vi "EditRowValue.vi"(0 "VI Reference In":refnum<vi>, 2 "delimiter (>>)":string=">>", 5 "Control Path":string, 7 "Row Index":i32, 9 "Value":string[](array[string]), 11 "Error In":errorcluster) -> (4 "VI Reference Out":refnum<vi>, 15 "Error Out":errorcluster)   [LabVIEW 2016, in "Drona.lvlib" / "ControlValue.lvlib" / "StimulusTable.lvlib"]
doc: "Sets value(signaling) for the table control whose row index is specified. \n\nThe input control name is given as a string , incase of path, use delimiters inbetween the path."
uses:
  StimulusTable.lvlib
  <vilib>/Utility/error.llb/Error Cluster From Error Code.vi
  <vilib>/ErrorRing/Error Ring.xnode
  Drona.lvlib
  Get/GetControlRef/GetControlRef.lvlib
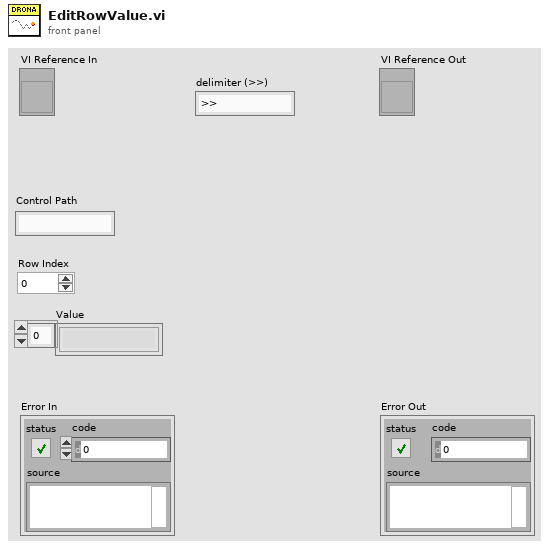
[diagram p1: front panel]
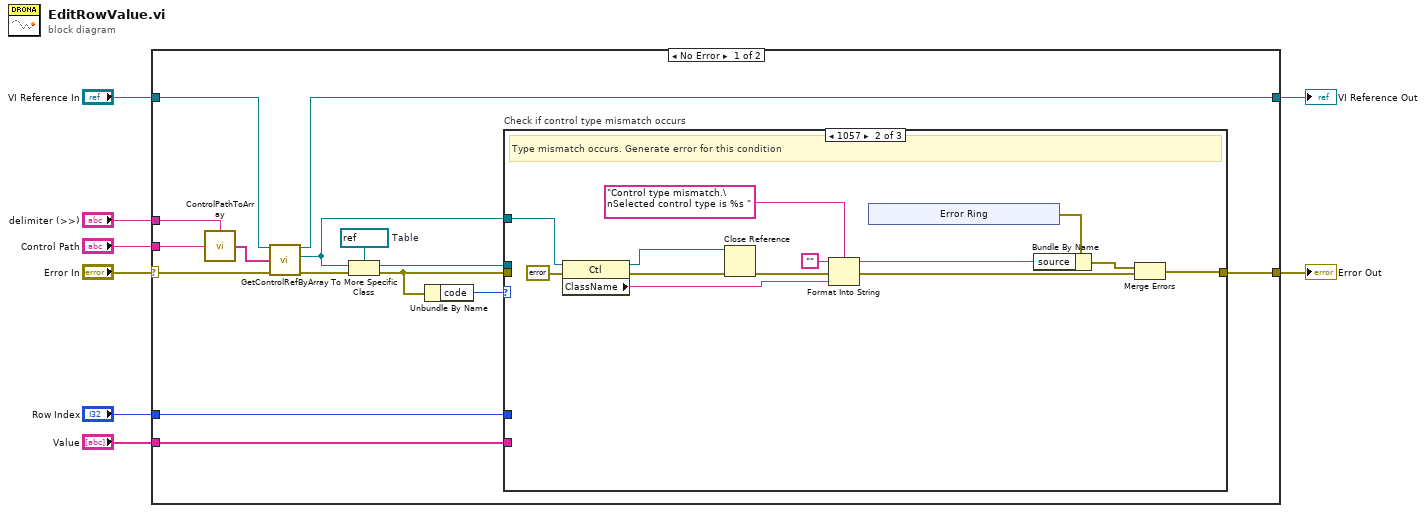
[diagram p0: block diagram]
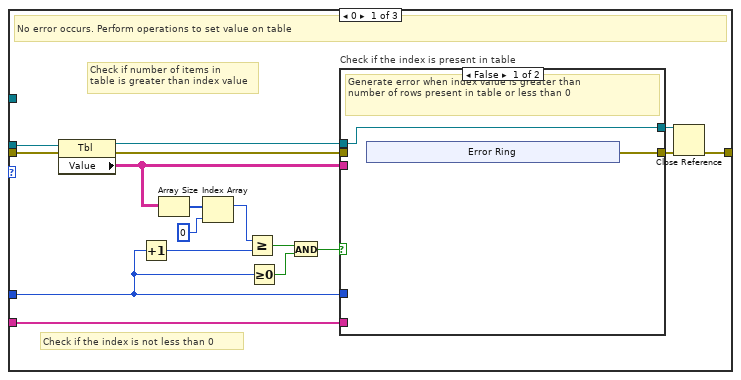
[diagram p2: hidden frame]
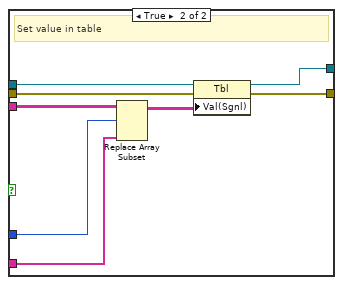
[diagram p3: hidden frame]
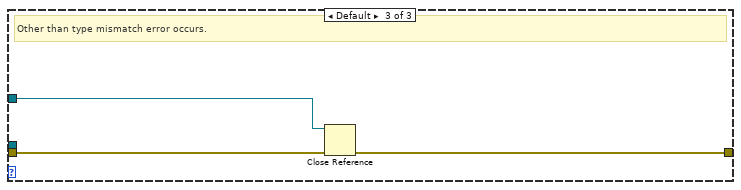
[diagram p4: hidden frame]
diagram:
  n1 = case shown="No Error" "Error In" {
    selector: "Error In" -> [w12 w78]
    tunnel: [w20 w78] -> w7
    tunnel: "VI Reference In" -> [w16 w77]
    tunnel: "Control Path" -> [w22 _]
    tunnel: "Row Index" -> [w18 _]
    tunnel: [w15 w77] -> w3
    tunnel: "delimiter (>>)" -> [w21 _]
    tunnel: "Value" -> [w9 _]
    frame No Error {
      w23 = refnum<vi> refnum  # Table
      n2 = call "ControlPathToArray.vi"("Control Name"=w22, "delimiter (>>)"=w21) -> ("Control Path"=w17:string[])
      n3 = call "GetControlRefByArray.vi"("VI Reference In"=w16, "Control Path"=w17, "error In"=w12) -> ("VI Reference Out"=w15:refnum<vi>, "Ctl Refnum"=w13:refnum<vi>, "error out"=w14:errorcluster)  [unwired: 10 in]
      n4 = To More Specific Class(target class=w23, reference=w13, error in=w14) -> (specific class reference=w19:refnum<vi>, error out=w11:errorcluster)
      n5 = Unbundle By Name(w11) -> ("code"=w10:i32)
      n6 = case "Check if control type mismatch occurs" shown="1057" w10 {
        tunnel: [w40 w58 w75] -> w20
        tunnel: w19 -> [w33 _ _]
        tunnel: w18 -> [w31 _ _]
        tunnel: w13 -> [_ w68 w74]
        tunnel: w11 -> [w39 _ w76]
        tunnel: w9 -> [w24 _ _]
        frame 0 {
          # "Check if number of items in \ntable is greater than index value"
          # "Check if the index is not less than 0"
          # "No error occurs. Perform operations to set value on table"
          n7 = property class="Tbl"(reference=w33, error in=w39) -> (reference out=w32:refnum<vi>, error out=w36:errorcluster, "Value"=w25:string[][])
          n8 = Increment(x=w31) -> (x+1=w34:i32)
          n9 = Array Size(array=w25) -> (size(s)=w35:i32[])
          n10 = Index Array(array=w35, index=0) -> (element=w27:i32)
          n11 = Greater Or Equal?(x=w27, y=w34) -> (x >= y?=w30:bool)
          n12 = Greater Or Equal To 0?(x=w31) -> (x >= 0?=w28:bool)
          n13 = And(x=w30, y=w28) -> (x .and. y?=w29:bool)
          n14 = case "Check if the index is present in table" shown="False" w29 {
            tunnel: [w41 w54] -> w38
            tunnel: [w42 w49] -> w37
            tunnel: w36 -> [_ w55]
            tunnel: w32 -> [w42 w53]
            tunnel: w31 -> [_ w48]
            tunnel: w25 -> [_ w52]
            tunnel: w24 -> [_ w50]
            frame False {
              # "Generate error when index value is greater than \nnumber of rows present in table or less than 0"
              n15 = xnode "Error Ring"() -> ("error out"=w41:errorcluster)
            }
            frame True {
              # "Set value in table"
              n16 = Replace Array Subset(array=w52, new element=w50, index (row)=w48) -> (w51:string[][])  [unwired: 1 in]
              n17 = property class="Tbl"(reference=w53, error in=w55, "Val(Sgnl)"=w51) -> (reference out=w49:refnum<vi>, error out=w54:errorcluster)
            }
          }
          n18 = Close Reference(reference=w37, error in (no error)=w38) -> (error out=w40:errorcluster)
        }
        frame 1057 {
          # "Type mismatch occurs. Generate error for this condition"
          n19 = property class="Ctl"(reference=w68, error in=errorcluster {"status"=FALSE, "code"=0, "source"=""} ("error out")) -> (reference out=w56:refnum<vi>, error out=w67:errorcluster, "ClassName"=w64:string)
          n20 = Close Reference(reference=w56, error in (no error)=w67) -> (error out=w57:errorcluster)
          n21 = Format Into String(format string="Control type mismatch.\nSelected control type is %s ", initial string="", error in=w57, w64) -> (resulting string=w61:string, error out=w59:errorcluster)
          n22 = xnode "Error Ring"() -> ("error out"=w62:errorcluster)
          n23 = Bundle By Name(cluster=w62, "source"=w61) -> (w60:errorcluster)
          n24 = Merge Errors(w60, w59) -> (w58:errorcluster)
        }
        frame Default {
          # "Other than type mismatch error occurs."
          n25 = Close Reference(reference=w74, error in (no error)=w76) -> (error out=w75:errorcluster)
        }
      }
    }
    frame Error {
    }
  }
  "Error Out" <- w7
  "VI Reference Out" <- w3
